vi "NewMazeGame.vi"(8 "error in (no error)":errorcluster) -> (0 "error out":errorcluster, 3 "MazeGame":refnum<class "MazeGame.lvclass">)   [LabVIEW 2020, in "FactoryMethod.lvlib" / "ParameterizedFactoryMethod.lvlib" / "MazeGame.lvclass"]
uses:
  MazeGame.lvclass
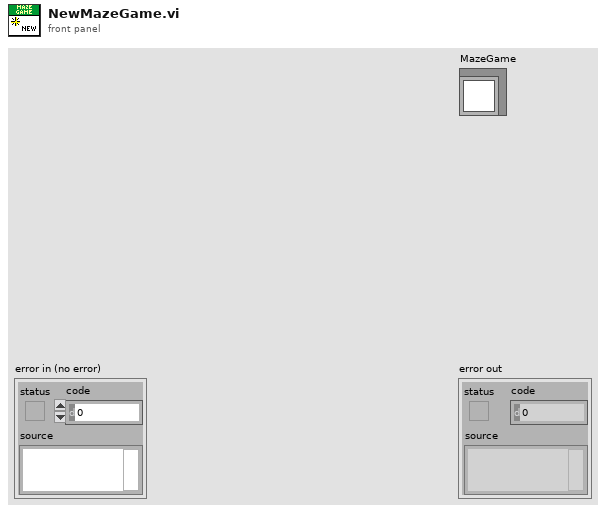
[diagram p1: front panel]
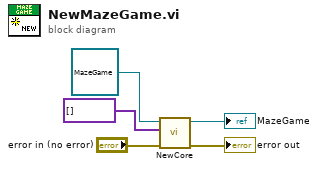
[diagram p0: block diagram]
diagram:
  n1 = call-dynamic "NewCore.vi"("error in (no error)"="error in (no error)", "ParamsArray"=variant[] [], "MazeGame"=refnum<class "MazeGame.lvclass"> refnum ("ByRef")) -> ("error out"=→"error out":errorcluster, "MazeGame"=→"MazeGame":refnum<class "MazeGame.lvclass">)  [unwired: 7 in]
